vi "SG_WriteMeans.vi"(8 "error in":errorcluster, 11 "Mean":dbl[](array[numeric])) -> (0 "error out":errorcluster)   [LabVIEW 2016]
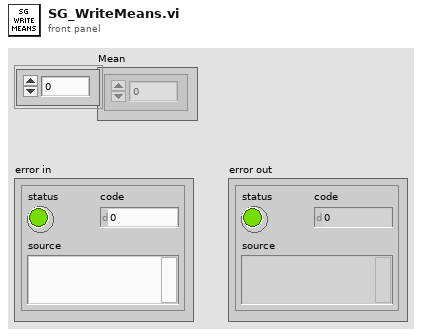
[diagram p1: front panel]
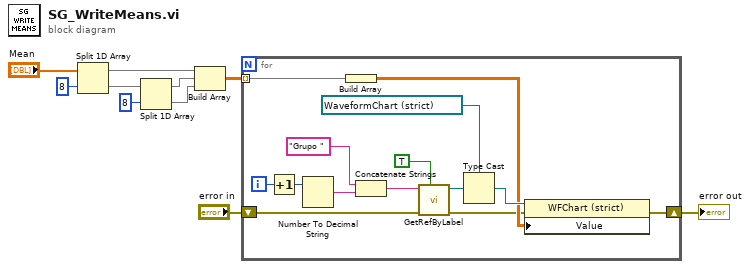
[diagram p0: block diagram]
diagram:
  n1 = Split 1D Array(array="Mean", index=8) -> (first subarray=w5:dbl[], second subarray=w6:dbl[])
  n2 = Split 1D Array(array=w6, index=8) -> (first subarray=w4:dbl[], second subarray=w3:dbl[])
  n3 = Build Array(w5, w4, w3) -> (w1:dbl[][])
  n4 = for {
    tunnel: w1 -> [w20] mode=indexing
    shift-right: [w22] -> w10
    shift-left: "error in" -> [w17]
    i -> [w15]
    n5 = Increment(x=w15) -> (x+1=w11:i32)
    n6 = Number To Decimal String(number=w11) -> (decimal integer string=w14:string)  [unwired: 1 in]
    n7 = Build Array(w20) -> (w19:dbl[][])
    n8 = Concatenate Strings("Grupo " ("Label"), w14) -> (w12:string)
    n9 = call "GetRefByLabel.vi"("InsideTab"=TRUE, "error in"=w17, "Label"=w12) -> ("error out"=w16:errorcluster, "Ctl Refnum"=w23:refnum<vi>)  [unwired: 6 in, 1 out]
    n10 = Type Cast(type=refnum<vi> refnum ("Grupo 1"), x=w23) -> (*(type *) &x=w21:refnum<vi>)
    n11 = property class="WFChart (strict)"(reference=w21, error in=w16, "Value"=w19) -> (error out=w22:errorcluster)  [unwired: 1 out]
  }
  "error out" <- w10
